vi "CRYUnary Operation Unit.vi"(6 "A _axis mode":u16(slide) scale=0.0..2.0, 8 "Unary Operator":u16(ring) items=["Change Sign", "Reciprocal Value", "Absolute Value", "Square", "Square Root", "Exp", "Ln", "Unwarp Phase", "Group Delay", "FFT", "Inverse FFT"], 9 "Type A":enum16{"Curves", "Values", "Results", "WFM"}(ring), 10 "Wave in":T1={"Waveform"={"X0"=0.0, "dX"=0.0, "Y"=[]}, "X data"=1, "Y data"=1, "Y axis"=1, "X unit"="s", "Y unit"="V", "Y dB ref"=1.0, "display Y"=TRUE, "display X"=TRUE, "Overload?"=FALSE, "Test Info"="", "Step No."=0, "Name"="", "protected"=FALSE, "Sqc history"=[], "Signal Channel ID"=0, "Plot Settings"={"Color"=0, "Interpolation"=0, "Point Style"=0, "Line Style"=0, "Point Color"=0, "Line Width"=0, "Bar Plot Style"=0, "Fill To"=0}, "AutoProtect"=FALSE} {"Y dB ref" format="%.1f"; "Y axis" items=["Log", "Lin"]; "Y data" items=["dB", "Lin"]; "X data" items=["dB", "Lin"]}, 11 "Operand A":T2={"Name"="", "Curve"=[], "X data"=1, "Y data"=1, "Z data"=1, "X axis"=0, "Y axis"=1, "Z axis"=1, "X unit"="Hz", "Y unit"="", "Z unit"="deg.", "X dB ref"=1.0, "Y dB ref"=1.0, "Z dB ref"=1.0, "single val"=FALSE, "protected"=FALSE, "display X"=TRUE, "display Y"=TRUE, "display Z"=TRUE, "Test Info"="", "Step No."=0, "Plot Settings"={"Color"=0, "Interpolation"=0, "Point Style"=0, "Line Style"=0, "Point Color"=0, "Line Width"=0, "Bar Plot Style"=0, "Fill To"=0}, "AutoProtect"=FALSE} {"Z data" items=["dB", "Lin"]; "X data" items=["dB", "Lin"]; "Y data" items=["dB", "Lin"]; "Z dB ref" format="%.1f"; "Z axis" items=["Log", "Lin"]; "X dB ref" format="%.1f"; "X axis" items=["Log", "Lin"]; "Y axis" items=["Log", "Lin"]; "Y dB ref" format="%.1f"; "Curve"."z" format="%.2f"; "Curve"."y" format="%.2f"; "Curve"."x" format="%.2f"}) -> (1 "Type out":enum16{"Curves", "Values", "Results", "WFM"}(ring), 2 "Wave out":T1={"Waveform"={"X0"=0.0, "dX"=0.0, "Y"=[]}, "X data"=1, "Y data"=1, "Y axis"=1, "X unit"="s", "Y unit"="V", "Y dB ref"=1.0, "display Y"=TRUE, "display X"=TRUE, "Overload?"=FALSE, "Test Info"="", "Step No."=0, "Name"="", "protected"=FALSE, "Sqc history"=[], "Signal Channel ID"=0, "Plot Settings"={"Color"=0, "Interpolation"=0, "Point Style"=0, "Line Style"=0, "Point Color"=0, "Line Width"=0, "Bar Plot Style"=0, "Fill To"=0}, "AutoProtect"=FALSE} {"Y dB ref" format="%.1f"; "Y axis" items=["Log", "Lin"]; "Y data" items=["dB", "Lin"]; "X data" items=["dB", "Lin"]}, 3 "Result":T2={"Name"="", "Curve"=[], "X data"=1, "Y data"=1, "Z data"=1, "X axis"=0, "Y axis"=1, "Z axis"=1, "X unit"="Hz", "Y unit"="", "Z unit"="deg.", "X dB ref"=1.0, "Y dB ref"=1.0, "Z dB ref"=1.0, "single val"=FALSE, "protected"=FALSE, "display X"=TRUE, "display Y"=TRUE, "display Z"=TRUE, "Test Info"="", "Step No."=0, "Plot Settings"={"Color"=0, "Interpolation"=0, "Point Style"=0, "Line Style"=0, "Point Color"=0, "Line Width"=0, "Bar Plot Style"=0, "Fill To"=0}, "AutoProtect"=FALSE} {"Z data" items=["dB", "Lin"]; "X data" items=["dB", "Lin"]; "Y data" items=["dB", "Lin"]; "Z dB ref" format="%.1f"; "Z axis" items=["Log", "Lin"]; "X dB ref" format="%.1f"; "X axis" items=["Log", "Lin"]; "Y axis" items=["Log", "Lin"]; "Y dB ref" format="%.1f"; "Curve"."z" format="%.2f"; "Curve"."y" format="%.2f"; "Curve"."x" format="%.2f"})   [LabVIEW 2013]
uses:
  Typedef Control/CRYData Cluster.ctl
  Typedef Control/CRYWaveform Cluster.ctl
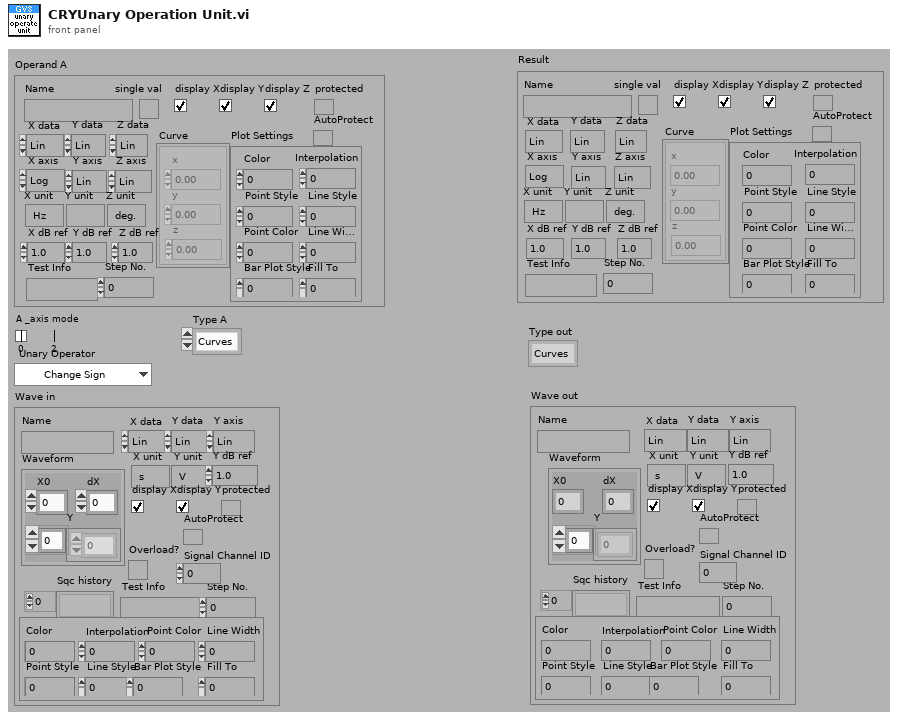
[diagram p1: front panel]
types:
  T1 = typedef "CRYWaveform Cluster.ctl" = cluster{"Waveform":cluster{"X0":dbl, "dX":dbl, "Y":sgl[]}, "X data":u16, "Y data":u16, "Y axis":u16, "X unit":string, "Y unit":string, "Y dB ref":dbl, "display Y":bool, "display X":bool, "Overload?":bool, "Test Info":string, "Step No.":i32, "Name":string, "protected":bool, "Sqc history":string[], "Signal Channel ID":i32, "Plot Settings":cluster{"Color":u32, "Interpolation":u8, "Point Style":u8, "Line Style":u8, "Point Color":u32, "Line Width":u8, "Bar Plot Style":u8, "Fill To":i16}, "AutoProtect":bool}
  T2 = typedef "CRYData Cluster.ctl" = cluster{"Name":string, "Curve":cluster{"x":dbl, "y":dbl, "z":dbl}[], "X data":u16, "Y data":u16, "Z data":u16, "X axis":u16, "Y axis":u16, "Z axis":u16, "X unit":string, "Y unit":string, "Z unit":string, "X dB ref":dbl, "Y dB ref":dbl, "Z dB ref":dbl, "single val":bool, "protected":bool, "display X":bool, "display Y":bool, "display Z":bool, "Test Info":string, "Step No.":i32, "Plot Settings":cluster{"Color":u32, "Interpolation":u8, "Point Style":u8, "Line Style":u8, "Point Color":u32, "Line Width":u8, "Bar Plot Style":u8, "Fill To":i16}, "AutoProtect":bool}
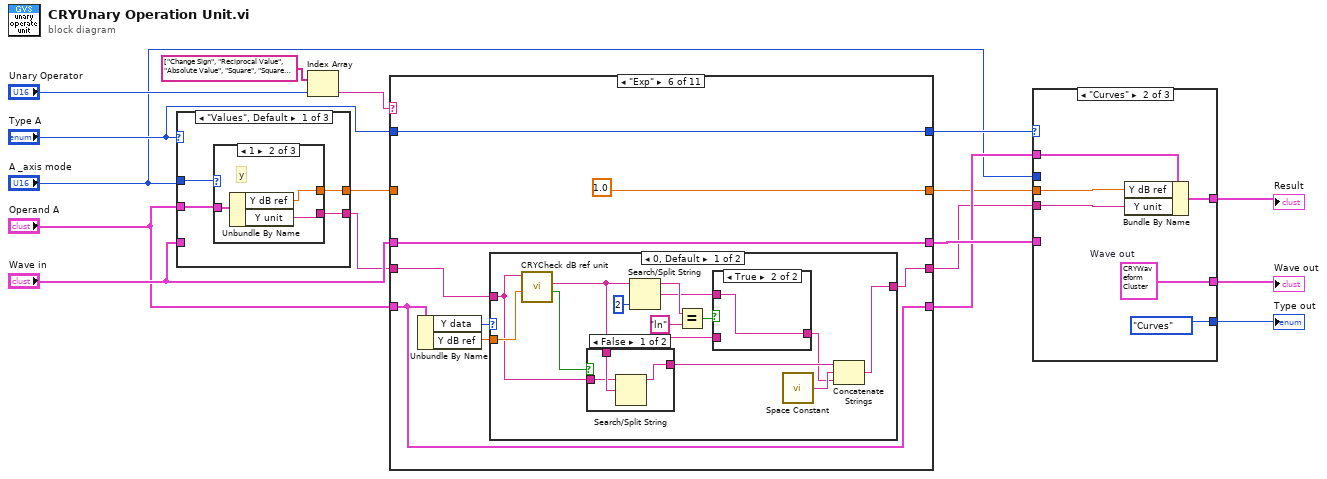
[diagram p0: block diagram]
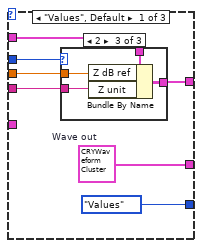
[diagram p2: hidden frame]
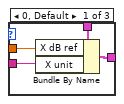
[diagram p3: hidden frame]
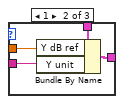
[diagram p4: hidden frame]
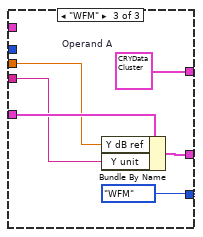
[diagram p5: hidden frame]
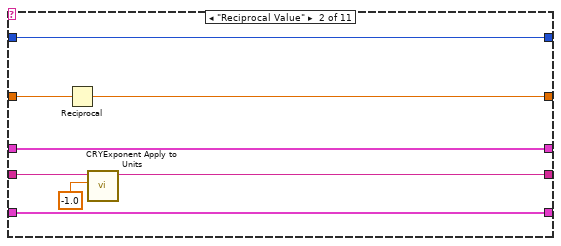
[diagram p7: hidden frame]
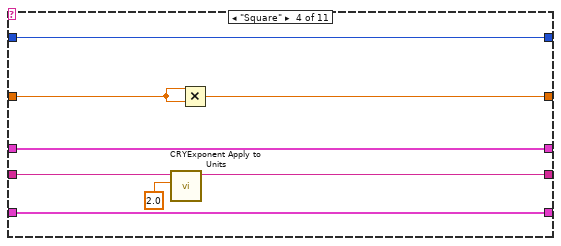
[diagram p9: hidden frame]
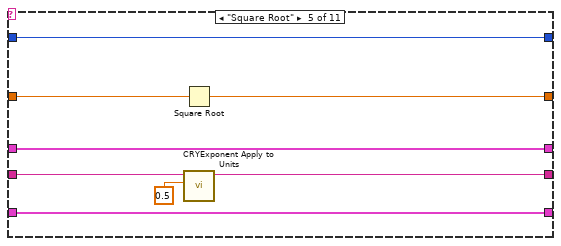
[diagram p10: hidden frame]
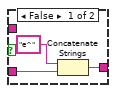
[diagram p12: hidden frame]
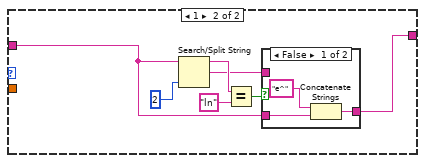
[diagram p13: hidden frame]
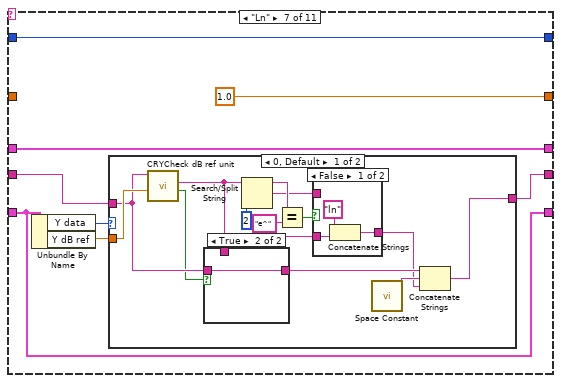
[diagram p15: hidden frame]
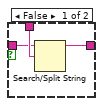
[diagram p16: hidden frame]
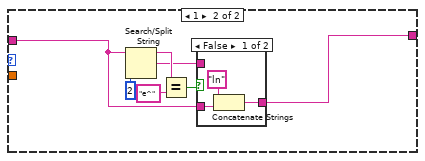
[diagram p18: hidden frame]
diagram:
  n1 = case shown="\"Values\", Default" "Type A" {
    tunnel: [w21 w33 w34] -> w11
    tunnel: [w18 w31 w35] -> w12
    tunnel: "Operand A" -> [w19 w32 _]
    tunnel: "A _axis mode" -> [w20 _ _]
    tunnel: "Wave in" -> [_ _ w36]
    frame "Values", Default {
      n2 = case shown="1" w20 {
        tunnel: w19 -> [w24 w27 w30]
        tunnel: [w23 w26 w29] -> w21
        tunnel: [w22 w25 w28] -> w18
        frame 0, Default {
          # "x"
          n3 = Unbundle By Name(w24) -> ("X dB ref"=w22:dbl, "X unit"=w23:string)
        }
        frame 1 {
          # "y"
          n4 = Unbundle By Name(w27) -> ("Y dB ref"=w25:dbl, "Y unit"=w26:string)
        }
        frame 2 {
          # "Z"
          n5 = Unbundle By Name(w30) -> ("Z dB ref"=w28:dbl, "Z unit"=w29:string)
        }
      }
    }
    frame "Curves" {
      n6 = Unbundle By Name(w32) -> ("Y dB ref"=w31:dbl, "Y unit"=w33:string)
    }
    frame "WFM" {
      n7 = Unbundle By Name(w36) -> ("Y dB ref"=w35:dbl, "Y unit"=w34:string)
    }
  }
  n8 = Index Array(array=string[] ["Change Sign", "Reciprocal Value", "Absolute Value", "Square", "Square Root", "Exp", "Ln", "Unwarp Phase", "Group Delay", "FFT", "Inverse FFT"] ("Unary Op Name"), index="Unary Operator") -> (element=w15:string)
  n9 = case shown="\"Exp\"" w15 {
    tunnel: w11 -> [w40 w47 w53 w60 w68 w75 w117 w154 _ w170 _]
    tunnel: w12 -> [w41 w49 w54 w62 w70 _ _ w155 w163 w169 w186]
    tunnel: [w41 w45 w54 w58 w66 1.0 1.0 w155 w163 w169 w186] -> w6
    tunnel: [w40 w46 w53 w59 w67 w78 w116 w154 "s" ("Y unit") w166 w178] -> w4
    tunnel: "Operand A" -> [w39 w44 w52 w57 w65 w73 w113 w153 w159 w167 w184]
    tunnel: [w39 w44 w52 w57 w65 w73 w113 w153 w156 w168 w184] -> w8
    tunnel: "Wave in" -> [w38 w43 w51 w56 w64 w72 w112 w152 w162 w165 w181]
    tunnel: [w38 w43 w51 w56 w64 w72 w112 w152 w162 w165 w179] -> w9
    tunnel: "Type A" -> [w37 w42 w50 w55 w63 w71 w111 w151 w161 _ _]
    tunnel: [w37 w42 w50 w55 w63 w71 w111 w151 w161 enum16{"Curves", "Values", "Results", "WFM"}."Curves" ("Type A") enum16{"Curves", "Values", "Results", "WFM"}."WFM" ("Type A")] -> w7
    frame "Change Sign", Default {
    }
    frame "Reciprocal Value" {
      n10 = Reciprocal(x=w49) -> (1/x=w45:dbl)
      n11 = call "CRYExponent Apply to Units.vi"("Exponent to apply"=-1.0, "Unit in"=w47) -> ("Unit out"=w46:string)  [unwired: 9 out]
    }
    frame "Absolute Value" {
    }
    frame "Square" {
      n12 = call "CRYExponent Apply to Units.vi"("Exponent to apply"=2.0, "Unit in"=w60) -> ("Unit out"=w59:string)  [unwired: 9 out]
      n13 = Multiply(x=w62, y=w62) -> (x*y=w58:dbl)
    }
    frame "Square Root" {
      n14 = Square Root(x=w70) -> (sqrt(x)=w66:dbl)
      n15 = call "CRYExponent Apply to Units.vi"("Exponent to apply"=0.5, "Unit in"=w68) -> ("Unit out"=w67:string)  [unwired: 9 out]
    }
    frame "Exp" {
      n16 = Unbundle By Name(w73) -> ("Y data"=w76:u16, "Y dB ref"=w74:dbl)
      n17 = case shown="0, Default" w76 {
        tunnel: [w82 w106] -> w78
        tunnel: w75 -> [w84 w100]
        tunnel: w74 -> [w86 _]
        frame 0, Default {
          n18 = call "CRYCheck dB ref unit.vi"("dB ref in"=w86, "Unit in"=w84) -> ("dB ref N/dB ref N **?"=w79:bool, "Lin unit out"=w85:string)  [unwired: 8 out]
          n19 = case shown="False" w79 {
            tunnel: w85 -> [w94 _]
            tunnel: w84 -> [w93 w95]
            tunnel: [w92 w95] -> w83
            frame False {
              n20 = Search/Split String(string=w93, search string/char (-)=w94) -> (substring before match=w92:string)  [unwired: 3 out]
            }
            frame True {
            }
          }
          n21 = Search/Split String(string=w85, offset (0)=2) -> (substring before match=w89:string, match + rest of string=w87:string)  [unwired: 2 out]
          n22 = Equal?(x=w89, y="ln") -> (x = y?=w88:bool)
          n23 = case shown="True" w88 {
            tunnel: w85 -> [w98 _]
            tunnel: [w96 w99] -> w80
            tunnel: w87 -> [_ w99]
            frame False {
              n24 = Concatenate Strings("e^", w98) -> (w96:string)
            }
            frame True {
            }
          }
          n25 = call <vilib>:"Space Constant.vi"() -> ("String"=w81:string)
          n26 = Concatenate Strings(w83, w81, w80) -> (w82:string)
        }
        frame 1 {
          n27 = Search/Split String(string=w100, offset (0)=2) -> (substring before match=w103:string, match + rest of string=w101:string)  [unwired: 2 out]
          n28 = Equal?(x=w103, y="ln") -> (x = y?=w102:bool)
          n29 = case shown="False" w102 {
            tunnel: w100 -> [w109 _]
            tunnel: [w107 w110] -> w106
            tunnel: w101 -> [_ w110]
            frame False {
              n30 = Concatenate Strings("e^", w109) -> (w107:string)
            }
            frame True {
            }
          }
        }
      }
    }
    frame "Ln" {
      n31 = Unbundle By Name(w113) -> ("Y data"=w115:u16, "Y dB ref"=w114:dbl)
      n32 = case shown="0, Default" w115 {
        tunnel: w117 -> [w124 w141]
        tunnel: [w120 w140] -> w116
        tunnel: w114 -> [w131 _]
        frame 0, Default {
          n33 = call "CRYCheck dB ref unit.vi"("dB ref in"=w131, "Unit in"=w124) -> ("dB ref N/dB ref N **?"=w119:bool, "Lin unit out"=w125:string)  [unwired: 8 out]
          n34 = case shown="True" w119 {
            tunnel: w125 -> [w134 _]
            tunnel: w124 -> [w133 w135]
            tunnel: [w132 w135] -> w123
            frame False {
              n35 = Search/Split String(string=w133, search string/char (-)=w134) -> (substring before match=w132:string)  [unwired: 3 out]
            }
            frame True {
            }
          }
          n36 = Search/Split String(string=w125, offset (0)=2) -> (substring before match=w128:string, match + rest of string=w126:string)  [unwired: 2 out]
          n37 = Equal?(x=w128, y="e^") -> (x = y?=w127:bool)
          n38 = case shown="False" w127 {
            tunnel: w125 -> [w138 _]
            tunnel: [w136 w139] -> w121
            tunnel: w126 -> [_ w139]
            frame False {
              n39 = Concatenate Strings("ln", w138) -> (w136:string)
            }
            frame True {
            }
          }
          n40 = call <vilib>:"Space Constant.vi"() -> ("String"=w122:string)
          n41 = Concatenate Strings(w123, w122, w121) -> (w120:string)
        }
        frame 1 {
          n42 = Search/Split String(string=w141, offset (0)=2) -> (substring before match=w144:string, match + rest of string=w142:string)  [unwired: 2 out]
          n43 = Equal?(x=w144, y="e^") -> (x = y?=w143:bool)
          n44 = case shown="False" w143 {
            tunnel: w141 -> [w149 _]
            tunnel: [w147 w150] -> w140
            tunnel: w142 -> [_ w150]
            frame False {
              n45 = Concatenate Strings("ln", w149) -> (w147:string)
            }
            frame True {
            }
          }
        }
      }
    }
    frame "Unwarp Phase" {
    }
    frame "Group Delay" {
      n46 = Bundle By Name(cluster=w159, "Y data"=u16 1, "Z unit"="") -> (w156:T2)
    }
    frame "FFT" {
      n47 = Format Value(format string="%#p", value (0)=w169) -> (output string=w174:string)  [unwired: 1 in]
      n48 = Bundle By Name(cluster=w167, "X unit"="Hz", "Y data"=u16 0) -> (w168:T2)
      n49 = call <vilib>:"Space Constant.vi"() -> ("String"=w175:string)
      n50 = Concatenate Strings("dB re" ("Y unit"), w175, w174, w175, w170) -> (w166:string)
    }
    frame "Inverse FFT" {
      w180 = "s" ("X unit")
      n51 = Unbundle By Name(w184) -> ("Y data"=w185:u16)
      n52 = case shown="0, Default" w185 {
        tunnel: w184 -> [w188 w192]
        tunnel: [w187 w191] -> w182
        frame 0, Default {
          n53 = Unbundle By Name(w188) -> ("Y unit"=w190:string, "Y dB ref"=w189:dbl)
          n54 = call "CRYCheck dB ref unit.vi"("dB ref in"=w189, "Unit in"=w190) -> ("Lin unit out"=w187:string)  [unwired: 6 in, 3 out]
        }
        frame 1 {
          n55 = Unbundle By Name(w192) -> ("Y unit"=w191:string)
        }
      }
      n56 = Concatenate Strings(w182, "/" ("string"), w180) -> (w178:string)
      n57 = Bundle By Name(cluster=w181, "X unit"=w180) -> (w179:T1)
    }
  }
  n58 = case shown="\"Curves\"" w7 {
    tunnel: w8 -> [w195 w215 _]
    tunnel: w6 -> [w199 w212 w220]
    tunnel: w4 -> [w198 w217 w219]
    tunnel: [w197 w216 w223] -> w3
    tunnel: "A _axis mode" -> [w196 _ _]
    tunnel: [enum16{"Curves", "Values", "Results", "WFM"}."Values" ("Type In") enum16{"Curves", "Values", "Results", "WFM"}."Curves" ("Type In") enum16{"Curves", "Values", "Results", "WFM"}."WFM" ("Type In")] -> w1
    tunnel: [w193 w213 w218] -> w2
    tunnel: w9 -> [_ _ w221]
    frame "Values", Default {
      w193 = T1 {"Waveform"={"X0"=0.0, "dX"=0.0, "Y"=[]}, "X data"=1, "Y data"=1, "Y axis"=1, "X unit"="s", "Y unit"="V", "Y dB ref"=1.0, "display Y"=TRUE, "display X"=TRUE, "Overload?"=FALSE, "Test Info"="", "Step No."=0, "Name"="", "protected"=FALSE, "Sqc history"=[], "Signal Channel ID"=0, "Plot Settings"={"Color"=0, "Interpolation"=0, "Point Style"=0, "Line Style"=0, "Point Color"=0, "Line Width"=0, "Bar Plot Style"=0, "Fill To"=0}, "AutoProtect"=FALSE}  # Wave out
      n59 = case shown="2" w196 {
        tunnel: w195 -> [w202 w207 w210]
        tunnel: w199 -> [w200 w204 w208]
        tunnel: w198 -> [w203 w205 w211]
        tunnel: [w201 w206 w209] -> w197
        frame 0, Default {
          n60 = Bundle By Name(cluster=w202, "X dB ref"=w200, "X unit"=w203) -> (w201:T2)
        }
        frame 1 {
          n61 = Bundle By Name(cluster=w207, "Y dB ref"=w204, "Y unit"=w205) -> (w206:T2)
        }
        frame 2 {
          n62 = Bundle By Name(cluster=w210, "Z dB ref"=w208, "Z unit"=w211) -> (w209:T2)
        }
      }
    }
    frame "Curves" {
      w213 = T1 {"Waveform"={"X0"=0.0, "dX"=0.0, "Y"=[]}, "X data"=1, "Y data"=1, "Y axis"=1, "X unit"="s", "Y unit"="V", "Y dB ref"=1.0, "display Y"=TRUE, "display X"=TRUE, "Overload?"=FALSE, "Test Info"="", "Step No."=0, "Name"="", "protected"=FALSE, "Sqc history"=[], "Signal Channel ID"=0, "Plot Settings"={"Color"=0, "Interpolation"=0, "Point Style"=0, "Line Style"=0, "Point Color"=0, "Line Width"=0, "Bar Plot Style"=0, "Fill To"=0}, "AutoProtect"=FALSE}  # Wave out
      n63 = Bundle By Name(cluster=w215, "Y dB ref"=w212, "Y unit"=w217) -> (w216:T2)
    }
    frame "WFM" {
      w223 = T2 {"Name"="", "Curve"=[], "X data"=1, "Y data"=1, "Z data"=1, "X axis"=0, "Y axis"=1, "Z axis"=1, "X unit"="Hz", "Y unit"="", "Z unit"="deg.", "X dB ref"=1.0, "Y dB ref"=1.0, "Z dB ref"=1.0, "single val"=FALSE, "protected"=FALSE, "display X"=TRUE, "display Y"=TRUE, "display Z"=TRUE, "Test Info"="", "Step No."=0, "Plot Settings"={"Color"=0, "Interpolation"=0, "Point Style"=0, "Line Style"=0, "Point Color"=0, "Line Width"=0, "Bar Plot Style"=0, "Fill To"=0}, "AutoProtect"=FALSE}  # Operand A
      n64 = Bundle By Name(cluster=w221, "Y dB ref"=w220, "Y unit"=w219) -> (w218:T1)
    }
  }
  "Result" <- w3
  "Wave out" <- w2
  "Type out" <- w1
